vi "布尔条件结构.vi"() -> ()   [LabVIEW 2022 SP3]
doc: "本VI是为《我和LabVIEW》一书编写的示例。\n关于本书的介绍请参考网页：\nhttp://ruanqizhen.spaces.live.com/blog/cns!5852D4F797C53FB6!4310.entry"
panel:
  in  "数值":dbl
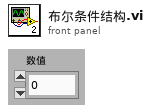
[diagram p1: front panel]
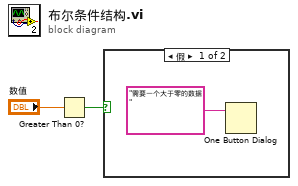
[diagram p0: block diagram]
diagram:
  n1 = Greater Than 0?(x="数值") -> (x > 0?=w1:bool)
  n2 = case shown="假" w1 {
    frame False {
      n3 = One Button Dialog(message="需要一个大于零的数据") -> ()  [unwired: 2 out]
    }
    frame True {
    }
  }
